vi "4031V3Project.vi"() -> ()   [LabVIEW 2024]
uses:
  <vilib>/Utility/TradDaqScaling.llb/Convert Thermocouple Reading (array).vi
  <vilib>/Utility/file.llb/Write Delimited Spreadsheet (DBL).vi
  <vilib>/Utility/file.llb/Write Delimited Spreadsheet (string).vi
  <vilib>/Analysis/NI_AALBase.lvlib
panel:
  out "Hot Out":sgl[](graph)
  out "Hot in":sgl[](graph)
  out "Tco Std":dbl
  out "Tci Std":dbl
  out "Tho Std":dbl
  out "Thi SD":dbl
  out "Hot side Delta":dbl format="%#_13g"
  out "Cold Side Delta":dbl format="%#_13g"
  in  "Sampling rate":dbl
  in  "Number of Samples":dbl
  out "Tco Mean":dbl
  out "Tci Mean":dbl
  out "Tho Mean":dbl
  out "Thi Mean":dbl
  out "Cold Out":sgl[](graph)
  out "Cold In":sgl[](graph)
  in  "?":bool
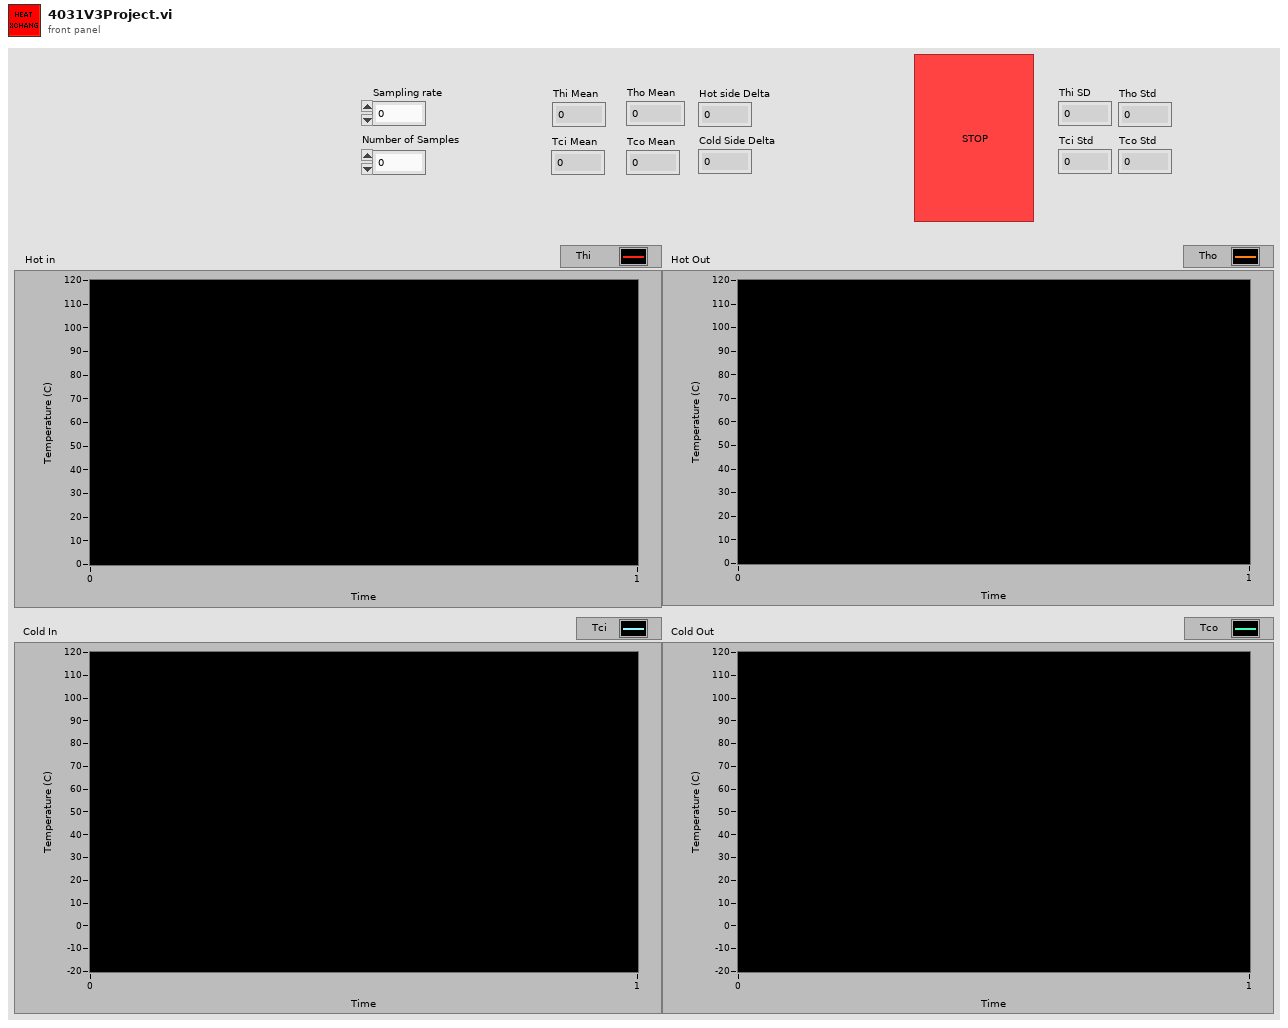
[diagram p1: front panel]
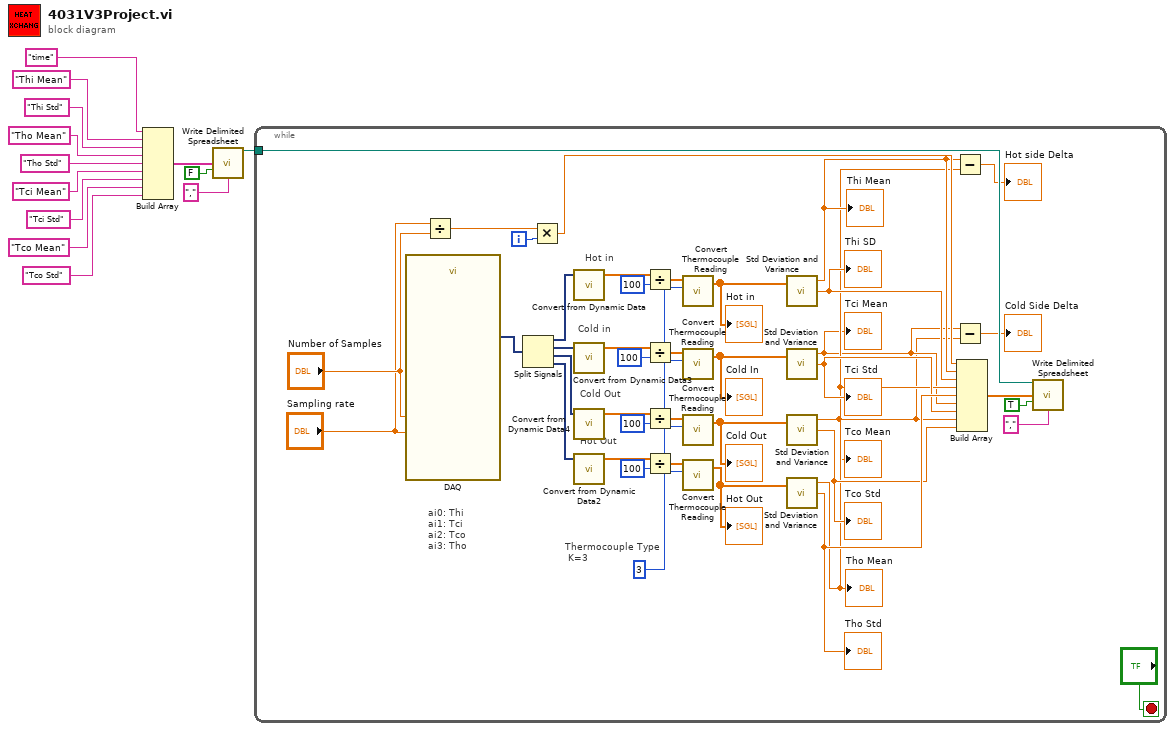
[diagram p0: block diagram]
diagram:
  n1 = Build Array("time", "Thi Mean", "Thi Std", "Tho Mean", "Tho Std", "Tci Mean", "Tci Std", "Tco Mean", "Tco Std") -> (w9:string[])
  n2 = call-poly <vilib>:"Write Delimited Spreadsheet.vi"("1D data"=w9, "append to file? (new file:F)"=FALSE, "delimiter (\\t)"=",") -> ("new file path (Not A Path if cancelled)"=w7:path)  [unwired: 11 in, 1 out]
  n3 = while {
    tunnel: w7 -> [w51]
    i -> [w39]
    stop <- "?" stop-if-true
    w14 = 3
    # "ai0: Thi\nai1: Tci\nai2: Tco\nai3: Tho"
    # "Thermocouple Type\n K=3"
    # "Hot Out"
    # "Cold Out"
    # "Cold in"
    # "Hot in"
    n4 = call "DAQ"("rate"="Sampling rate", "number of samples"="Number of Samples") -> ("data"=w19:dynamicdata)  [unwired: 15 in, 2 out]
    n5 = Divide(x="Sampling rate", y="Number of Samples") -> (x/y=w47:dbl)
    n6 = Split Signals(w19) -> (w18:dynamicdata, w17:dynamicdata, w16:dynamicdata, w15:dynamicdata)  [unwired: 4 in]
    n7 = Multiply(x=w47, y=w39) -> (x*y=w35:dbl)
    n8 = call "Convert from Dynamic Data"("Dynamic Data Type"=w18) -> ("Array"=w49:dbl[])  [unwired: 3 in]
    n9 = call "Convert from Dynamic Data3"("Dynamic Data Type"=w17) -> ("Array"=w38:dbl[])  [unwired: 3 in]
    n10 = call "Convert from Dynamic Data4"("Dynamic Data Type"=w16) -> ("Array"=w37:dbl[])  [unwired: 3 in]
    n11 = call "Convert from Dynamic Data2"("Dynamic Data Type"=w15) -> ("Array"=w45:dbl[])  [unwired: 3 in]
    n12 = Divide(x=w49, y=100) -> (x/y=w48:dbl[])
    n13 = Divide(x=w38, y=100) -> (x/y=w42:dbl[])
    n14 = Divide(x=w37, y=100) -> (x/y=w40:dbl[])
    n15 = Divide(x=w45, y=100) -> (x/y=w44:dbl[])
    n16 = call-poly <vilib>:"Convert Thermocouple Reading.vi"("ThermocoupleType"=w14, "Voltage Array"=w48) -> ("Temperature Array"=w29:sgl[])  [unwired: 5 in]
    "Hot in" <- w29
    n17 = call-poly <vilib>:"Convert Thermocouple Reading.vi"("ThermocoupleType"=w14, "Voltage Array"=w42) -> ("Temperature Array"=w27:sgl[])  [unwired: 5 in]
    "Cold In" <- w27
    n18 = call-poly <vilib>:"Convert Thermocouple Reading.vi"("ThermocoupleType"=w14, "Voltage Array"=w40) -> ("Temperature Array"=w26:sgl[])  [unwired: 5 in]
    "Cold Out" <- w26
    n19 = call-poly <vilib>:"Convert Thermocouple Reading.vi"("ThermocoupleType"=w14, "Voltage Array"=w44) -> ("Temperature Array"=w28:sgl[])  [unwired: 5 in]
    "Hot Out" <- w28
    n20 = call <vilib>:"Std Deviation and Variance.vi"("X"=w29) -> ("mean"=w23:dbl, "standard deviation"=w36:dbl)  [unwired: 1 in, 1 out]
    "Thi Mean" <- w23
    "Thi SD" <- w36
    n21 = call <vilib>:"Std Deviation and Variance.vi"("X"=w27) -> ("mean"=w21:dbl, "standard deviation"=w33:dbl)  [unwired: 1 in, 1 out]
    "Tci Mean" <- w21
    "Tci Std" <- w33
    n22 = call <vilib>:"Std Deviation and Variance.vi"("X"=w26) -> ("mean"=w20:dbl, "standard deviation"=w32:dbl)  [unwired: 1 in, 1 out]
    "Tco Mean" <- w20
    "Tco Std" <- w32
    n23 = call <vilib>:"Std Deviation and Variance.vi"("X"=w28) -> ("mean"=w22:dbl, "standard deviation"=w34:dbl)  [unwired: 1 in, 1 out]
    "Tho Mean" <- w22
    "Tho Std" <- w34
    n24 = Subtract(x=w23, y=w22) -> (x-y=→"Hot side Delta":dbl)
    n25 = Subtract(x=w21, y=w20) -> (x-y=→"Cold Side Delta":dbl)
    n26 = Build Array(w35, w23, w36, w22, w34, w21, w33, w20, w32) -> (w53:dbl[])
    n27 = call-poly <vilib>:"Write Delimited Spreadsheet.vi"("file path (dialog if empty)"=w51, "1D data"=w53, "append to file? (new file:F)"=TRUE, "delimiter (\\t)"=",") -> ()  [unwired: 10 in, 2 out]
  }
